vi "ReadConfigFile.vi"(8 "error in (no error)":errorcluster, 11 "Microscope_RM21 in":refnum<class "Microscope_RM21.lvclass">) -> (0 "error out":errorcluster, 3 "Microscope_RM21 out":refnum<class "Microscope_RM21.lvclass">)   [LabVIEW 2020, in "Microscope_RM21.lvlib" / "Microscope_RM21.lvclass"]
uses:
  Microscope_RM21.lvclass
  <vilib>/Utility/config.llb/Read Key (I32).vi
  Hardware Abstraction Layer/Microscope/Microscope/Microscope.lvclass
  <vilib>/Utility/config.llb/NI_LVConfig.lvlib
panel:
  out "s? t:f":i32
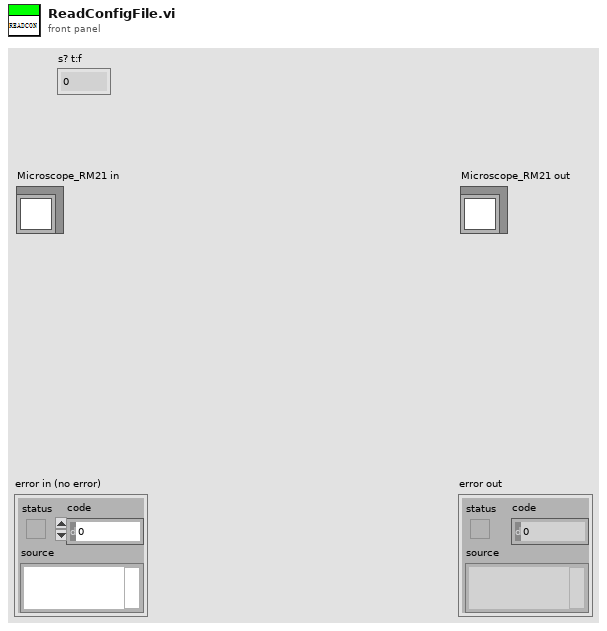
[diagram p1: front panel]
types:
  T1 = typedef "NI_LVConfig.lvlib/Config Data RefNum.ctl" = refnum<k1>
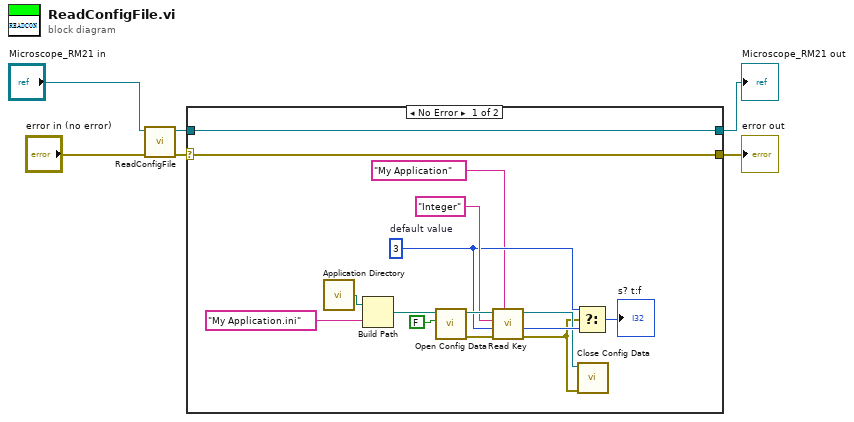
[diagram p0: block diagram]
diagram:
  n1 = call-parent "ReadConfigFile.vi"("error in (no error)"="error in (no error)", "Device in"="Microscope_RM21 in") -> ("error out"=w4:errorcluster, "Device out"=w3:refnum<class "Microscope_RM21.lvclass">)  [unwired: 8 in]
  n2 = case shown="No Error" w4 {
    selector: w4 -> [w10 w23]
    tunnel: [w10 w23] -> w1
    tunnel: [w8 w22] -> w2
    tunnel: w3 -> [w8 w22]
    frame No Error {
      w14 = 3  # default value
      n3 = call <vilib>:"Application Directory.vi"() -> ("Application Directory"=w21:path)
      n4 = Build Path(base path=w21, name or relative path="My Application.ini") -> (appended path=w19:path)
      n5 = call <vilib>:"Open Config Data.vi"("create file if necessary (T)"=FALSE, "configuration file path"=w19) -> ("error out"=w17:errorcluster, "refnum"=w16:T1)  [unwired: 7 in, 1 out]
      n6 = call-poly <vilib>:"Read Key.vi"("section"="My Application", "error in (no error)"=w17, "default value"=w14, "key"="Integer", "refnum"=w16) -> ("error out"=w11:errorcluster, "value"=w13:i32, "refnum out"=w12:T1)  [unwired: 3 in, 1 out]
      n7 = Select(t=w14, s=w11, f=w13) -> (s? t:f=→"s? t:f":i32)
      n8 = call <vilib>:"Close Config Data.vi"("error in (no error)"=w11, "refnum"=w12) -> ()  [unwired: 8 in, 2 out]
    }
    frame Error {
    }
  }
  "error out" <- w1
  "Microscope_RM21 out" <- w2
